vi "RefreshDisplay.vi"(8 "error in (no error)":errorcluster, 11 "Serial Controller in":refnum<class "Serial Controller.lvclass">) -> (0 "error out":errorcluster, 3 "Serial Controller out":refnum<class "Serial Controller.lvclass">)   [LabVIEW 2010, in "Serial Controller.lvclass"]
uses:
  Serial Controller.lvclass
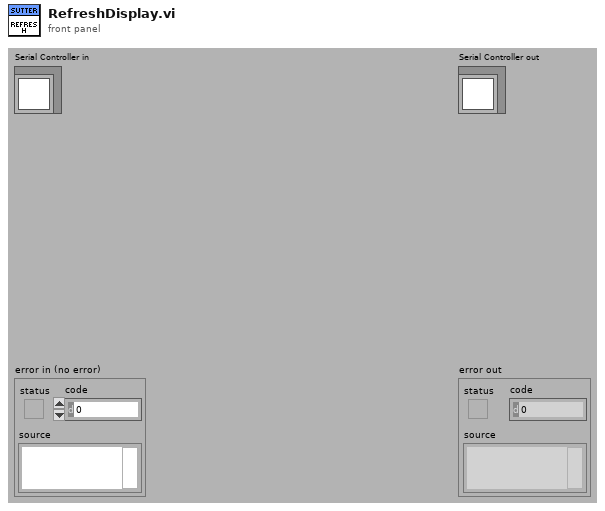
[diagram p1: front panel]
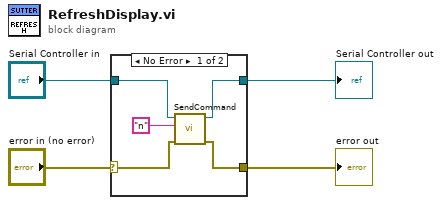
[diagram p0: block diagram]
diagram:
  n1 = case shown="No Error" "error in (no error)" {
    selector: "error in (no error)" -> [w8 w11]
    tunnel: [w5 w11] -> w3
    tunnel: [w6 w10] -> w1
    tunnel: "Serial Controller in" -> [w9 w10]
    frame No Error {
      n2 = call-dynamic "SendCommand.vi"("error in (no error)"=w8, "command"="n", "Serial Controller in"=w9) -> ("error out"=w5:errorcluster, "Serial Controller out"=w6:refnum<class "Serial Controller.lvclass">)  [unwired: 6 in, 1 out]
    }
    frame Error {
    }
  }
  "error out" <- w3
  "Serial Controller out" <- w1
